vi "ROI entry screen-LBox delete rows.vi"(8 "error in (no error)":errorcluster) -> (0 "error out":errorcluster)   [LabVIEW 2020]
uses:
  Typedefs/ROI management FG states.ctl
  Typedefs/Redraw ROI.ctl
  Typedefs/FGV ROI Time Ops.ctl
  Globals/gl_ROI Entry UI globals.vi
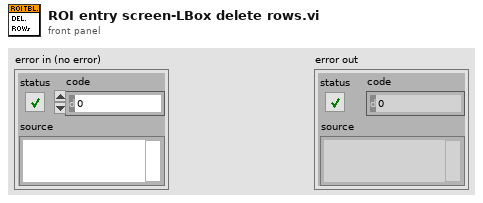
[diagram p1: front panel]
types:
  T1 = typedef "ROI entry screen ctrl refs cluster.ctl" = cluster{"Done button":refnum<vi>, "Imaging button":refnum<vi>, "Acquisition button":refnum<vi>, "Scan dwell time per pixel (us)":refnum<vi>, "# of planes":refnum<vi>, "Zoom Ctrl":refnum<vi>, "Equal size":refnum<vi>, "Channel":refnum<vi>, "Image Display":refnum<vi>, "Z-Plane Selector":refnum<vi>, "Number of lines left":refnum<vi>, "Z-stack folder path":refnum<vi>, "POI Density":refnum<vi>, "Arb Plane Entry":refnum<vi>, "Whole Plane":refnum<vi>, "Line Mode":refnum<vi>, "Clear Last":refnum<vi>, "Clear All":refnum<vi>, "Delete Lines":refnum<vi>, "Trial Length (sec)":refnum<vi>, "Palette Type":refnum<vi>, "Intensity slider":refnum<vi>, "# POI":refnum<vi>, "Max Z Proj":refnum<vi>, "Zplane ind":refnum<vi>, "Wavelength (nm)":refnum<vi>, "Number of Trials":refnum<vi>, "Funct stim.trig.enable":refnum<vi>, "Funct stim.trig.delay (s)":refnum<vi>, "Line Mode":refnum<vi>, "Step size (µm)":refnum<vi>, "ROI move mode":refnum<vi>, "Cool-down time (s)":refnum<vi>, "Enable cool-down time":refnum<vi>, "Motor Z ind. (um)":refnum<vi>, "AOL Z ind. (um)":refnum<vi>, "Load Reference Image":refnum<vi>, "Rel.  Res.":refnum<vi>, "ROI LIST":refnum<vi>, "Show All":refnum<vi>, "ROI Type":refnum<vi>, "Start Plane":refnum<vi>, "Stop Plane":refnum<vi>, "Offset ROI":refnum<vi>, "Tab Control":refnum<vi>, "Laser Power(%)":refnum<vi>, "Cycle rate":refnum<vi>, "FOV (Ind.)":refnum<vi>, "Frame Size (Ind.)":refnum<vi>, "Resolution (Ind.)":refnum<vi>, "Pixel Density (Ind)":refnum<vi>, "Laser Power (Ind.)":refnum<vi>, "Dwell Time (Ind.)":refnum<vi>, "Adj MC":refnum<vi>}
  T2 = typedef "FGV ROI Time Ops.ctl" = enum16{"Read", "Write Cycle Time", "Write Cycle Rate"}
  T3 = typedef "Redraw ROI.ctl" = enum16{"Redraw All", "Redraw Deselected", "Draw Last", "Redraw Selected"}
  T4 = typedef "ROI management FG states.ctl" = enum16{"Read", "Write", "Write-from dataset", "Clear Last", "Clear All", "Delete ROI", "Update ROIs time", "Reload last ROI set", "Modify ROI Parameters", "Offset all ROI", "Offset visible ROI", "Modify Dwell Time", "Modify Laser Power"}
  T5 = typedef "ROI parameters data type.ctl" = cluster{"ROI index":dbl, "ROI ID":dbl, "ROI Time (ns)":dbl, "Pixels in ROI":dbl, "X start":dbl, "Y start":dbl, "Z start":dbl, "X stop":dbl, "Y stop":dbl, "Z stop":dbl, "Angle (deg)":dbl, "Composite ID":dbl, "Number of lines":dbl, "Frame Size":dbl, "Zoom":dbl, "Laser Power (%)":dbl, "ROI group ID":dbl, "Resolution":dbl, "Dwell Time per pixel":dbl, "Pixels per miniscan":dbl, "Original FOV (um)":dbl, "Apparent Frame Size":dbl, "Z Plane Idx":i32[], "Z Plane codes":i32[]}
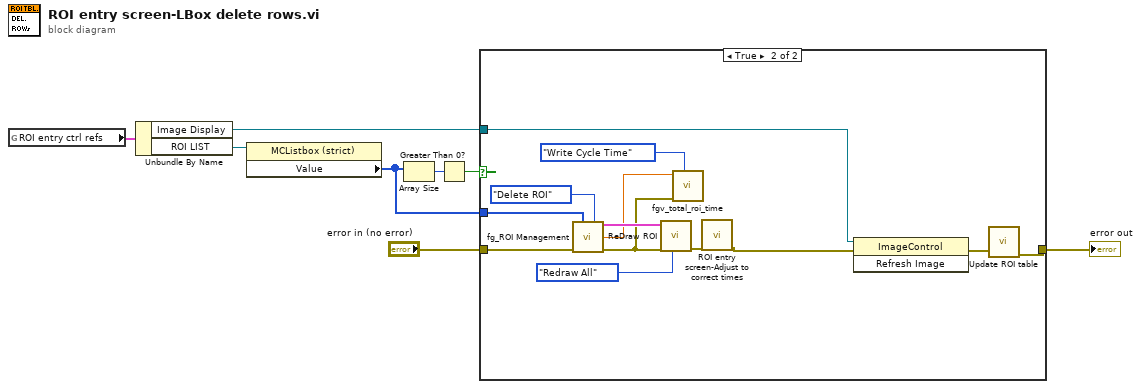
[diagram p0: block diagram]
diagram:
  n1 = global read "gl_ROI Entry UI globals.vi" "ROI entry ctrl refs"() -> (w2:T1)
  n2 = Unbundle By Name(w2) -> ("Image Display"=w1:refnum<vi>, "ROI LIST"=w8:refnum<vi>)
  n3 = property class="MCListbox (strict)"(reference=w8) -> ("Value"=w3:i32[])  [unwired: 1 in, 2 out]
  n4 = Array Size(array=w3) -> (size(s)=w7:i32)
  n5 = Greater Than 0?(x=w7) -> (x > 0?=w6:bool)
  n6 = case shown="True" w6 {
    tunnel: "error in (no error)" -> [w9 w22]
    tunnel: [w9 w17] -> w4
    tunnel: w3 -> [_ w18]
    tunnel: w1 -> [_ w16]
    frame False {
    }
    frame True {
      n7 = call "fg_ROI Management.vi"("ROIs for deletion"=w18, "Function"=ROI_management_FG_states."Delete ROI", "error in (no error)"=w22) -> ("ROI Setup"=w14:T5[], "Total ROI time"=w11:dbl, "error out"=w12:errorcluster)  [unwired: 6 in, 4 out]
      n8 = call "ReDraw ROI.vi"("Mode (Redraw All)"=Redraw_ROI."Redraw All", "error in"=w12, "XYZ Coordinates"=w14) -> ("error out"=w21:errorcluster)  [unwired: 8 in]
      n9 = call "fgv_total_roi_time.vi"("Op"=FGV_ROI_Time_Ops."Write Cycle Time", "error in (no error)"=w12, "Total cycle time"=w11) -> ()  [unwired: 4 in, 5 out]
      n10 = call "ROI entry screen-Adjust to correct times.vi"("error in (no error)"=w21) -> ("error out"=w13:errorcluster)  [unwired: 9 in, 1 out]
      n11 = invoke class="ImageControl" method="Refresh Image"(reference=w16, error in=w13) -> (error out=w15:errorcluster)  [unwired: 1 in, 2 out]
      n12 = call "Update ROI table.vi"("error in (no error)"=w15) -> ("error out"=w17:errorcluster)  [unwired: 10 in]
    }
  }
  "error out" <- w4
